vi "Controller Response and Correction Matrices Selection.vi"(9 "Correction  Matrices":dbl[][][](array[numeric]), 10 "Response Matrices":dbl[][][](array[numeric]), 11 "selected":i32) -> (1 "Selected Correction Matrix":dbl[][](array[numeric]), 2 "Selected Response Matrix":dbl[][](array[numeric]))   [LabVIEW 2011, in "Controller VIs.lvlib"]
uses:
  Controller VIs.lvlib
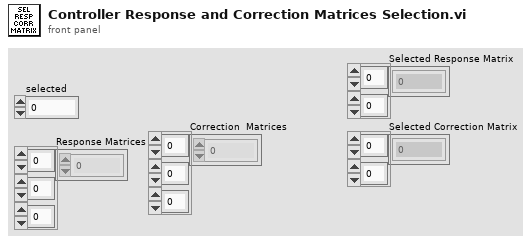
[diagram p1: front panel]
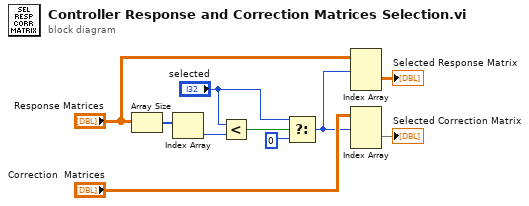
[diagram p0: block diagram]
diagram:
  n1 = Array Size(array="Response Matrices") -> (size(s)=w6:i32[])
  n2 = Index Array(array=w6) -> (element=w7:i32)  [unwired: 1 in]
  n3 = Less?(x="selected", y=w7) -> (x < y?=w8:bool)
  n4 = Select(t="selected", s=w8, f=0) -> (s? t:f=w3:i32)
  n5 = Index Array(array="Response Matrices", index (dim 0)=w3) -> (element=→"Selected Response Matrix":dbl[][])  [unwired: 2 in]
  n6 = Index Array(array="Correction  Matrices", index (dim 0)=w3) -> (element=→"Selected Correction Matrix":dbl[][])  [unwired: 2 in]
